vi "Get Paths.vi"(8 "error in (no error)":errorcluster, 11 "FP-TC-Shared in":refnum<class "FP-TC-Shared.lvclass">) -> (0 "error out":errorcluster, 2 "Paths":string[](array[string]), 3 "FP-TC-Shared out":refnum<class "FP-TC-Shared.lvclass">)   [LabVIEW 2019, in "FP-TC-Shared.lvclass"]
uses:
  FP-TC-Shared.lvclass
  FP-TC-Shared.lvclass/FP-TC-Shared.ctl
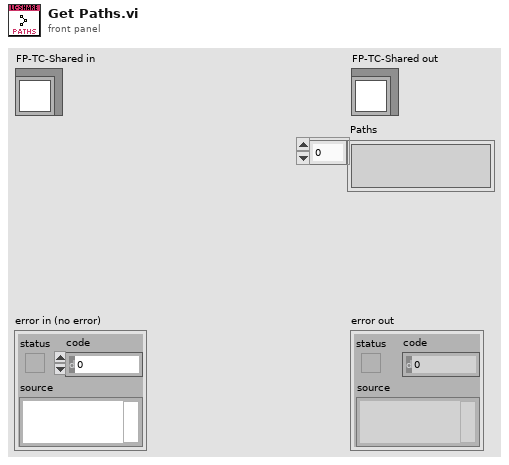
[diagram p1: front panel]
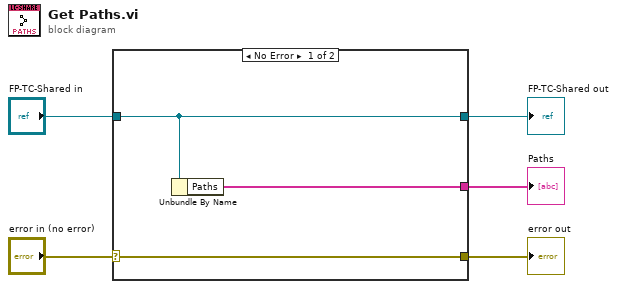
[diagram p0: block diagram]
diagram:
  n1 = case shown="No Error" "error in (no error)" {
    selector: "error in (no error)" -> [w7 w10]
    tunnel: [w8 _] -> w5
    tunnel: "FP-TC-Shared in" -> [w6 w9]
    tunnel: [w7 w10] -> w2
    tunnel: [w6 w9] -> w1
    frame No Error {
      n2 = Unbundle By Name(w6) -> ("Paths"=w8:string[])
    }
    frame Error {
    }
  }
  "error out" <- w2
  "FP-TC-Shared out" <- w1
  "Paths" <- w5
